vi "Write Filter settings.vi"(8 "error in (no error)":errorcluster, 10 "Filter settings":T1={"Decimation Scale (1-10)"=3, "Spatial Alpha\n(0-1)"=0.6, "Spatial Delta \n(1/32 disp)"=8, "Temporal Alpha\n(0-1)"=0.4, "Temporal Delta\n(1/32 disp)"=20, "Persistence (0= none, 8=max)"=0, "spatial holefill radius\n(0 disable, 5 max) "=0, "spatial iteration\n(2=default)"=2} {"spatial iteration\n(2=default)" min=1 max=10; "Decimation Scale (1-10)" min=1 max=10; "Spatial Alpha\n(0-1)" min=0 max=1 format="%_2g"; "Spatial Delta \n(1/32 disp)" min=1; "Temporal Alpha\n(0-1)" min=0 max=1 format="%_2g"; "Temporal Delta\n(1/32 disp)" min=1; "Persistence (0= none, 8=max)" max=8; "spatial holefill radius\n(0 disable, 5 max)" max=6}, 11 "Realsense Cam in":refnum<class "Realsense Cam.lvclass">) -> (0 "error out":errorcluster, 3 "Realsense Cam out":refnum<class "Realsense Cam.lvclass">)   [LabVIEW 2018, in "Realsense Cam.lvclass"]
uses:
  Realsense Cam.lvclass
  Realsense Cam.lvclass/Realsense Cam.ctl
  realsense_wrapper_api/libRealSense3.lvlib
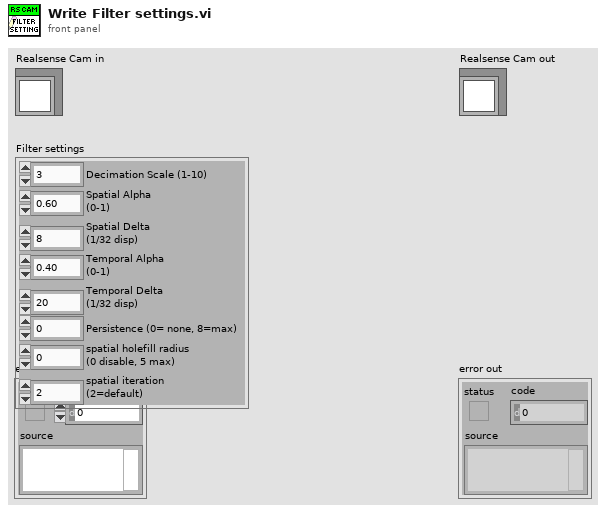
[diagram p1: front panel]
types:
  T1 = cluster{"Decimation Scale (1-10)":u8, "Spatial Alpha\n(0-1)":sgl, "Spatial Delta \n(1/32 disp)":u16, "Temporal Alpha\n(0-1)":sgl, "Temporal Delta\n(1/32 disp)":u16, "Persistence (0= none, 8=max)":u8, "spatial holefill radius\n(0 disable, 5 max) ":u8, "spatial iteration\n(2=default)":u8}
  T2 = cluster{"decimation filter block":u64, "spatial filter block":u64, "temporal filter block":u64, "disparity_transforg_2_block":u64, "disparity_transforg_1_block":u64}
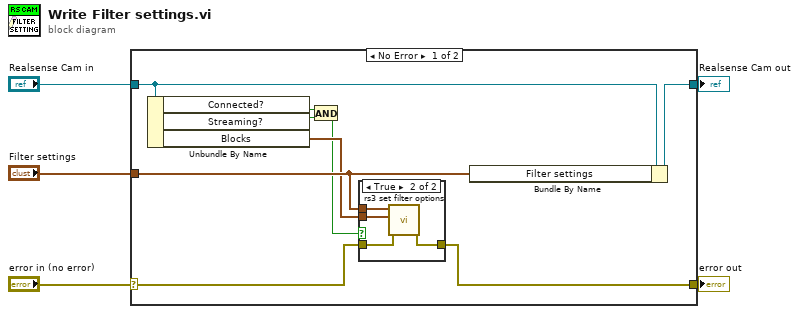
[diagram p0: block diagram]
diagram:
  n1 = case shown="No Error" "error in (no error)" {
    selector: "error in (no error)" -> [w7 w20]
    tunnel: [w6 w20] -> w4
    tunnel: [w14 w21] -> w2
    tunnel: "Realsense Cam in" -> [w12 w21]
    tunnel: "Filter settings" -> [w13 _]
    frame No Error {
      n2 = Unbundle By Name(w12) -> ("Connected?"=w9:bool, "Streaming?"=w10:bool, "Blocks"=w11:T2)
      n3 = And(x=w9, y=w10) -> (x .and. y?=w8:bool)
      n4 = case shown="True" w8 {
        tunnel: w13 -> [_ w19]
        tunnel: w11 -> [_ w18]
        tunnel: w7 -> [w15 w17]
        tunnel: [w15 w16] -> w6
        frame False {
        }
        frame True {
          n5 = call "rs3 set filter options.vi"("error in (no error)"=w17, "Processing Blocks"=w18, "Filter settings"=w19) -> ("error out"=w16:errorcluster)  [unwired: 8 in]
        }
      }
      n6 = Bundle By Name(cluster=w12, "Filter settings"=w13) -> (w14:refnum<class "Realsense Cam.lvclass">)
    }
    frame Error {
    }
  }
  "error out" <- w4
  "Realsense Cam out" <- w2
